vi "Acquisition Message Loop.vi"(0 "Message Queues":T2, 5 "Data Queue Logging":T1, 7 "Data Queue Processing":T1, 11 "error in (no error)":errorcluster) -> (15 "error out":errorcluster)   [LabVIEW 2021, in "IMU Acquisition.lvlib"]
doc: "Message loop for handling messages pertaining to the acquisition of data from the hardware."
uses:
  IMU Acquisition.lvlib
  support/Message Queue/All Message Queues.ctl
  support/Message Queue/Message Cluster.ctl
  IMU Data Queue.ctl
  IMU TimeDataStruct.ctl
  Hardware Configuration.ctl
  Settings/baudrates.ctl
  Acquisition State.ctl
  support/Message Queue/Enqueue Message (Single).vi
  <vilib>/Utility/error.llb/Error Cluster From Error Code.vi
  <vilib>/ErrorRing/Error Ring.xnode
  support/Message Queue/IMU Message Queue.lvlib
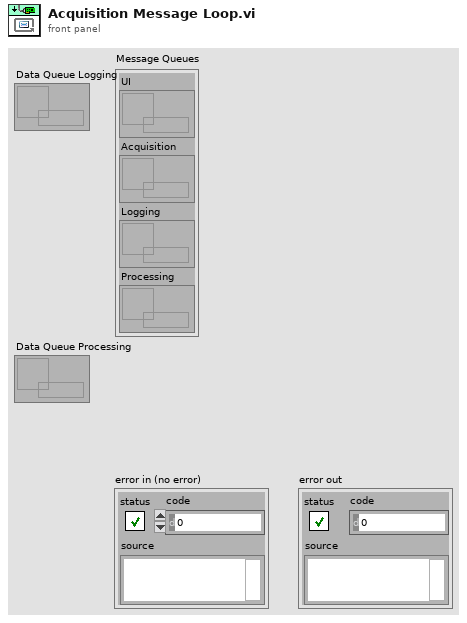
[diagram p1: front panel]
types:
  T1 = typedef "IMU Data Queue.ctl" = refnum<queue>
  T2 = typedef "IMU Message Queue.lvlib/All Message Queues.ctl" = cluster{"UI":refnum<queue>, "Acquisition":refnum<queue>, "Logging":refnum<queue>, "Processing":refnum<queue>}
  T3 = typedef "IMU Acquisition.lvlib/Hardware Configuration.ctl" = cluster{"Port":refnum<visa-resource-name>, "Baudrate":T4}
  T4 = typedef "baudrates.ctl" = u16
  T5 = typedef "IMU Acquisition.lvlib/Acquisition State.ctl" = enum16{"Flush", "Idle", "Acquiring"}
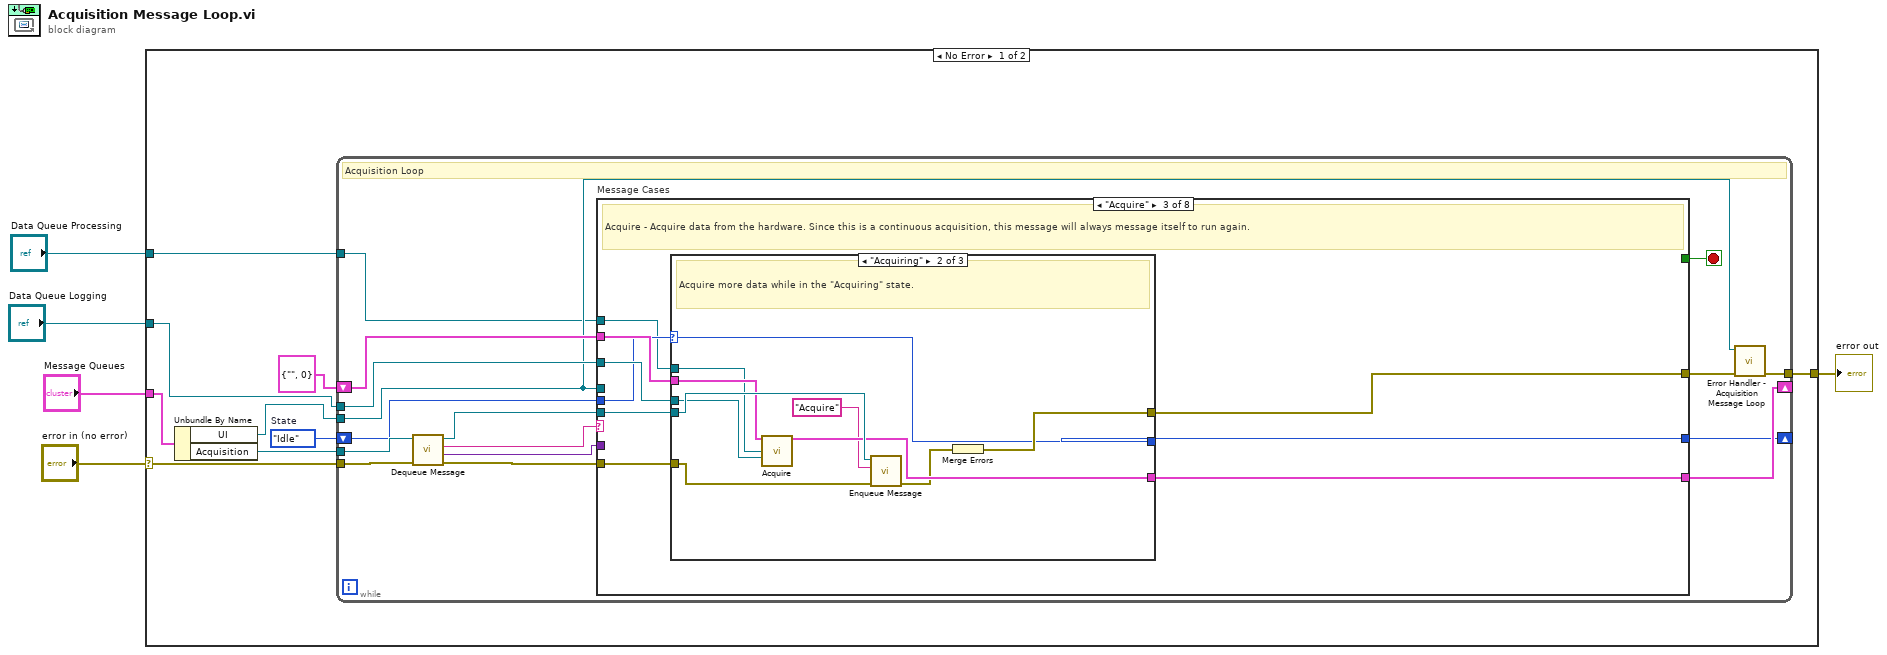
[diagram p0: block diagram]
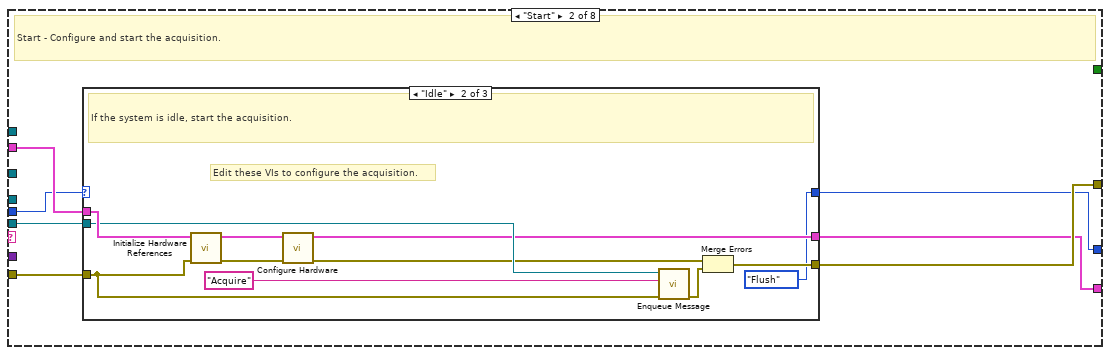
[diagram p3: hidden frame]
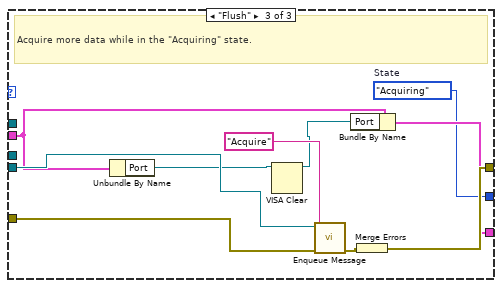
[diagram p7: hidden frame]
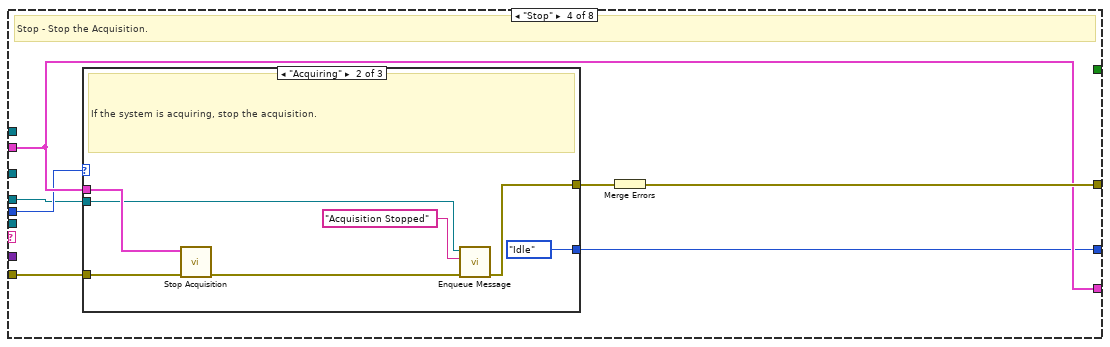
[diagram p8: hidden frame]
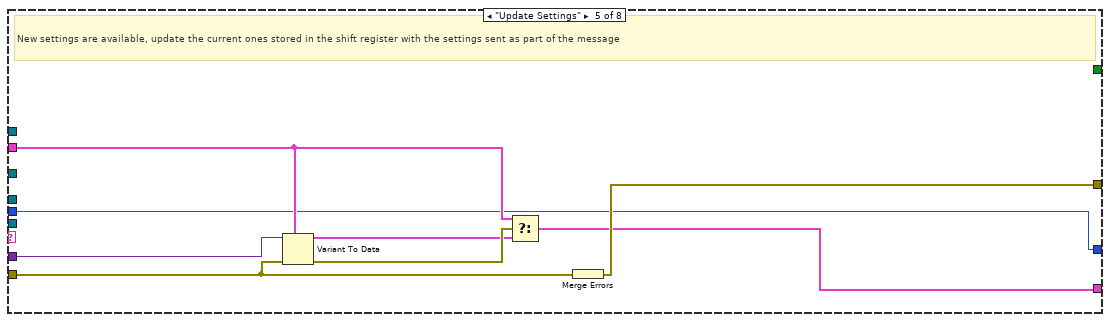
[diagram p11: hidden frame]
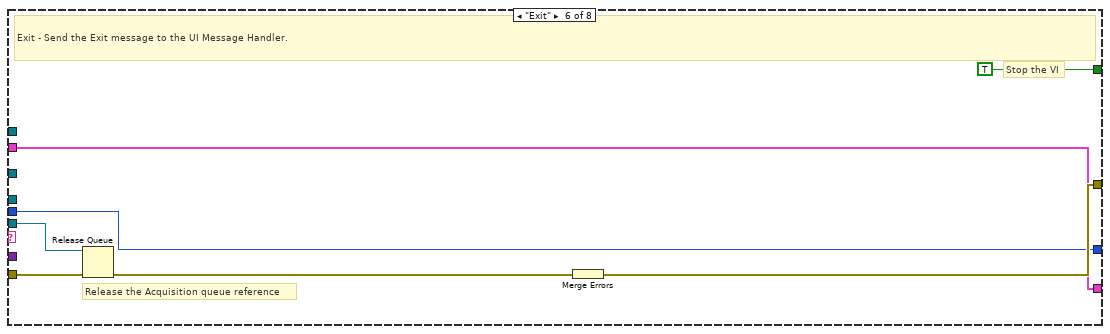
[diagram p12: hidden frame]
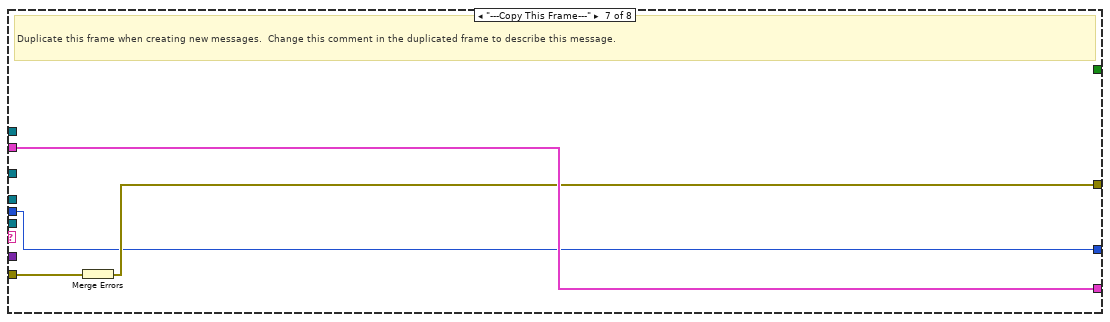
[diagram p13: hidden frame]
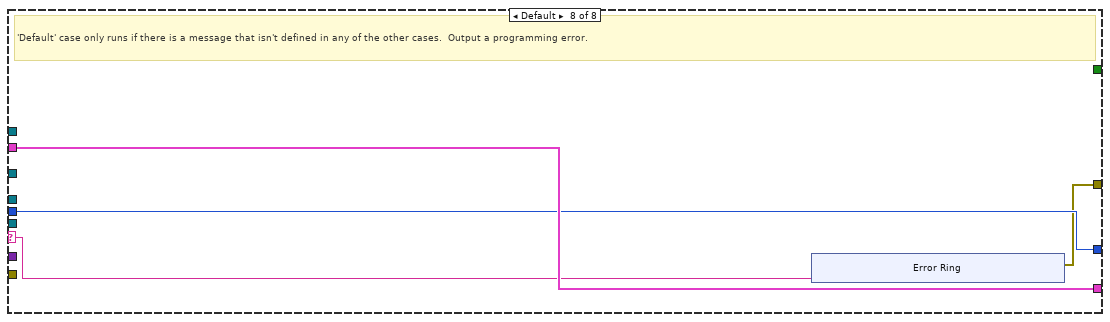
[diagram p14: hidden frame]
diagram:
  n1 = case shown="No Error" "error in (no error)" {
    selector: "error in (no error)" -> [w10 w138]
    tunnel: "Message Queues" -> [w14 _]
    tunnel: [w12 w138] -> w4
    tunnel: "Data Queue Logging" -> [w8 _]
    tunnel: "Data Queue Processing" -> [w6 _]
    frame No Error {
      w7 = Acquisition_State."Idle"  # State
      n2 = Unbundle By Name(w14) -> ("UI"=w9:refnum<queue>, "Acquisition"=w13:refnum<queue>)
      n3 = while {
        tunnel: w13 -> [w23]
        shift-right: [w29] -> _
        shift-left: T3 {"Port"="", "Baudrate"=0} ("Data Cluster") -> [w30]
        tunnel: w9 -> [w16]
        tunnel: w8 -> [w22]
        shift-right: [w20] -> _
        shift-left: w7 -> [w21]
        tunnel: w10 -> [w27]
        tunnel: [w19] -> w12
        tunnel: w6 -> [w15]
        stop <- w28 stop-if-true
        # "Acquisition Loop"
        n4 = call "Dequeue Message.vi"("error in (no error)"=w27, "Message Queue"=w23) -> ("error out"=w26:errorcluster, "Message Data"=w24:variant, "Message"=w25:string, "dup Message Queue"=w17:refnum<queue>)  [unwired: 6 in]
        n5 = case "Message Cases" shown="\"Acquire\"" w25 {
          selector: w25 -> [_ _ _ _ _ _ _ w127]
          tunnel: w17 -> [_ w37 w65 _ _ w117 _ _]
          tunnel: w26 -> [w33 w38 w64 w95 w109 w119 w126 _]
          tunnel: [w33 w40 w66 w96 w115 w121 w124 w128] -> w18
          tunnel: w30 -> [w32 w39 w62 w93 w111 w120 w125 w130]
          tunnel: [w32 w36 w63 w93 w110 w120 w125 w130] -> w29
          tunnel: [_ _ _ _ _ TRUE _ _] -> w28
          tunnel: w24 -> [_ _ _ _ w114 _ _ _]
          tunnel: w16 -> [_ _ _ w90 _ _ _ _]
          tunnel: w22 -> [_ _ w61 _ _ _ _ _]
          tunnel: w21 -> [w31 w34 w59 w92 w108 w116 w123 w129]
          tunnel: [w31 w35 w60 w91 w108 w116 w123 w129] -> w20
          tunnel: w15 -> [_ _ w58 _ _ _ _ _]
          frame "Initialize" {
            # "Initialize  - Initialize is currently a no-op.  The hardware initialization takes place in the 'Start' message."
          }
          frame "Start" {
            # "Start - Configure and start the acquisition."
            n6 = case shown="\"Idle\"" w34 {
              selector: w34 -> [w41 _ w55]
              tunnel: [w42 w54 w57] -> w40
              tunnel: w39 -> [w43 w53 w56]
              tunnel: w38 -> [w42 w52 w57]
              tunnel: w37 -> [_ w50 _]
              tunnel: [w43 w46 w56] -> w36
              tunnel: [w41 Acquisition_State."Flush" ("Acquisition State") w55] -> w35
              frame "Acquiring" {
                # "The system is already acquiring. Ignore the \"Start\" message."
              }
              frame "Idle" {
                # "Edit these VIs to configure the acquisition."
                # "If the system is idle, start the acquisition."
                n7 = call "Initialize Hardware References.vi"("error in (no error)"=w52, "Hardware Resources in"=w53) -> ("error out"=w49:errorcluster, "Hardware Resources out"=w47:T3)  [unwired: 8 in]
                n8 = call "Configure Hardware.vi"("error in (no error)"=w49, "Hardware Resources in"=w47) -> ("error out"=w48:errorcluster, "Hardware Resources out"=w46:T3)  [unwired: 8 in]
                n9 = call-poly "Enqueue Message.vi"("error in (no error)"=w52, "Message"="Acquire", "Message Queue"=w50) -> ("error out"=w51:errorcluster)  [unwired: 7 in, 1 out]
                n10 = Merge Errors(w48, w51) -> (w54:errorcluster)
              }
              frame "Flush" {
              }
            }
          }
          frame "Acquire" {
            # "Acquire - Acquire data from the hardware. Since this is a continuous acquisition, this message will always message itself to run again."
            n11 = case shown="\"Acquiring\"" w59 {
              selector: w59 -> [w67 w73 _]
              tunnel: [w68 w79 w89] -> w66
              tunnel: w65 -> [_ w78 w87]
              tunnel: w64 -> [w68 w71 w83]
              tunnel: [w69 w77 w85] -> w63
              tunnel: w62 -> [w69 w76 w84]
              tunnel: w61 -> [_ w74 _]
              tunnel: [w67 w73 w82] -> w60
              tunnel: w58 -> [_ w72 _]
              frame "Idle" {
                # "Ignore \"Acquire\" messages when the acquisition is idle."
              }
              frame "Acquiring" {
                # "Acquire more data while in the \"Acquiring\" state."
                n12 = call "Acquire.vi"("Hardware Resources in"=w76, "Data Queue Processing"=w72, "Data Queue Logging"=w74) -> ("Hardware Resources out"=w77:T3)  [unwired: 11 in, 1 out]
                n13 = call-poly "Enqueue Message.vi"("error in (no error)"=w71, "Message"="Acquire", "Message Queue"=w78) -> ("error out"=w70:errorcluster)  [unwired: 7 in, 1 out]
                n14 = Merge Errors(w70) -> (w79:errorcluster)
              }
              frame "Flush" {
                w82 = Acquisition_State."Acquiring"  # State
                # "Acquire more data while in the \"Acquiring\" state."
                n15 = Unbundle By Name(w84) -> ("Port"=w81:refnum<visa-resource-name>)
                n16 = VISA Clear(VISA resource name=w81) -> (VISA resource name out=w80:refnum<visa-resource-name>)  [unwired: 1 in, 1 out]
                n17 = call-poly "Enqueue Message.vi"("error in (no error)"=w83, "Message"="Acquire", "Message Queue"=w87) -> ("error out"=w88:errorcluster)  [unwired: 7 in, 1 out]
                n18 = Bundle By Name(cluster=w84, "Port"=w80) -> (w85:T3)
                n19 = Merge Errors(w88) -> (w89:errorcluster)
              }
            }
          }
          frame "Stop" {
            # "Stop - Stop the Acquisition."
            n20 = case shown="\"Acquiring\"" w92 {
              selector: w92 -> [w97 _ w106]
              tunnel: w95 -> [w98 w105 w107]
              tunnel: [w98 w101 w107] -> w94
              tunnel: w93 -> [_ w103 _]
              tunnel: [w97 Acquisition_State."Idle" ("State") w106] -> w91
              tunnel: w90 -> [_ w100 _]
              frame "Idle" {
                # "The system is already idle. Ignore the \"Stop\" message."
              }
              frame "Acquiring" {
                # "If the system is acquiring, stop the acquisition."
                n21 = call "Stop Acquisition.vi"("error in (no error)"=w105, "Hardware Resources in"=w103) -> ("error out"=w104:errorcluster)  [unwired: 9 in]
                n22 = call-poly "Enqueue Message.vi"("error in (no error)"=w104, "Message"="Acquisition Stopped", "Message Queue"=w100) -> ("error out"=w101:errorcluster)  [unwired: 7 in, 1 out]
              }
              frame "Flush" {
              }
            }
            n23 = Merge Errors(w94) -> (w96:errorcluster)
          }
          frame "Update Settings" {
            # "New settings are available, update the current ones stored in the shift register with the settings sent as part of the message"
            n24 = Variant To Data(error in=w109, type=w111, Variant=w114) -> (data=w112:T3, error out=w113:errorcluster)
            n25 = Select(t=w111, s=w113, f=w112) -> (s? t:f=w110:T3)
            n26 = Merge Errors(w109) -> (w115:errorcluster)
          }
          frame "Exit" {
            # "Release the Acquisition queue reference"
            # "Stop the VI"
            # "Exit - Send the Exit message to the UI Message Handler."
            n27 = Release Queue(queue=w117, error in (no error)=w119) -> (error out=w118:errorcluster)  [unwired: 1 in, 2 out]
            n28 = Merge Errors(w118) -> (w121:errorcluster)
          }
          frame "---Copy This Frame---" {
            # "Duplicate this frame when creating new messages.  Change this comment in the duplicated frame to describe this message."
            n29 = Merge Errors(w126) -> (w124:errorcluster)
          }
          frame Default {
            # "'Default' case only runs if there is a message that isn't defined in any of the other cases.  Output a programming error."
            n30 = xnode "Error Ring"("parameter 0"=w127) -> ("error out"=w128:errorcluster)
          }
        }
        n31 = call "Error Handler - Acquisition Message Loop.vi"("error in (no error)"=w18, "Message Queue"=w16) -> ("dup error in"=w19:errorcluster)  [unwired: 8 in, 1 out]
      }
    }
    frame Error {
    }
  }
  "error out" <- w4
